vi "Wash Display.vi"(8 "error in (no error)":errorcluster, 11 "Message Queues":T1) -> (0 "error out":errorcluster)   [LabVIEW 2017]
uses:
  support/Message Queue/All Message Queues.ctl
  support/Message Queue/Message Cluster.ctl
  Entry Display Data.ctl
  Position Slider.ctl
  Wash Step Indicators.ctl
  <vilib>/ErrorRing/Error Ring.xnode
  support/Message Queue/Message Queue.lvlib
panel:
  out "Time Eclipse":dbl
  out "Wash Entry Display":bool
  out "Vehicle Position":bool
  out "Air Dry":bool
  out "Tire Shine Foam":bool
  out "Spot Free Rinse":bool
  out "Low Pressure  Wax":bool
  out "High Pressure Wash":bool
  out "Pre-soak":bool
  out "Bug Remover":bool
  out "Under Body Wash":bool
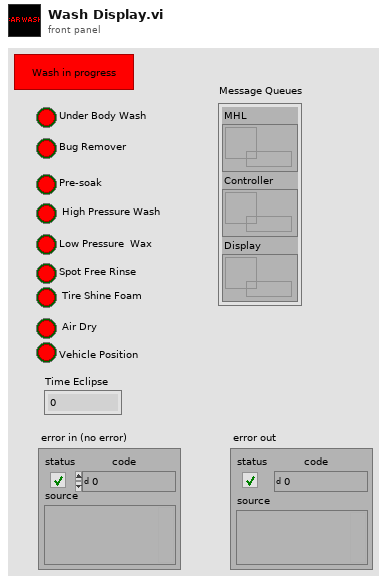
[diagram p1: front panel]
types:
  T1 = typedef "Message Queue.lvlib/All Message Queues.ctl" = cluster{"MHL":refnum<queue>, "Controller":refnum<queue>, "Display":refnum<queue>}
  T2 = typedef "Entry Display Data.ctl" = cluster{"Wash Entry Display":bool, "Car Position Slider":T3, "Wash Display Indicators":T4, "Vehicle Postion":bool}
  T3 = typedef "Position Slider.ctl" = i32
  T4 = typedef "Wash Step Indicators.ctl" = cluster{"Under Body Wash":bool, "Bug Remover":bool, "Pre-soak":bool, " High Pressure Wash":bool, "Low Pressure  Wax":bool, "Spot Free Rinse":bool, " Tire Shine Foam":bool, " Air Dry":bool}
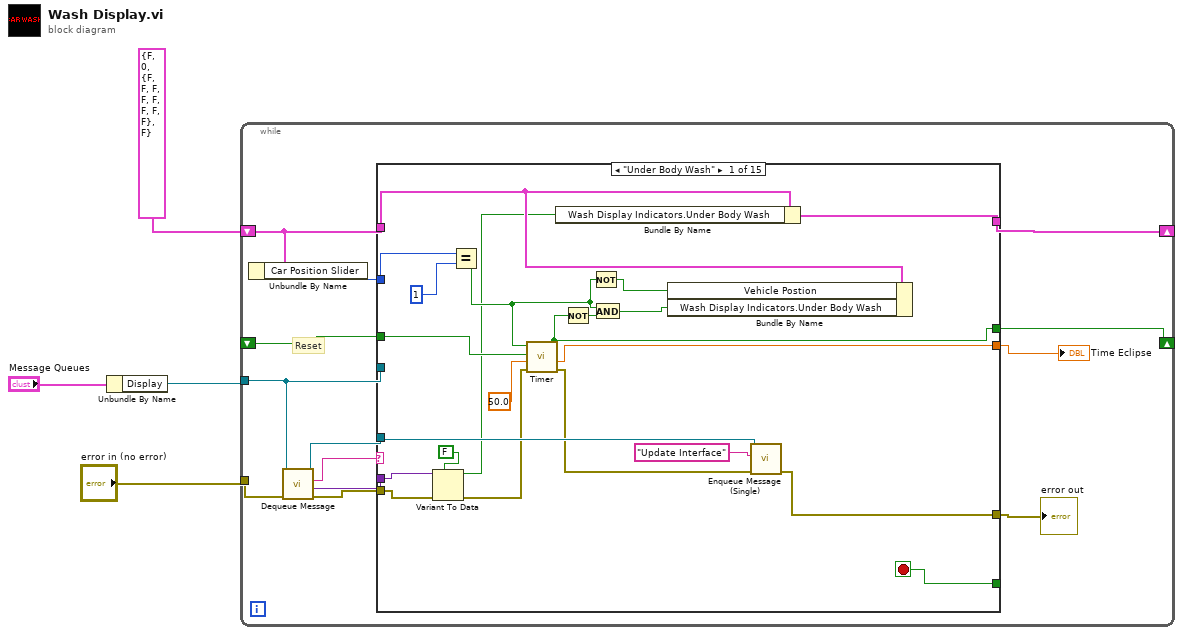
[diagram p0: block diagram]
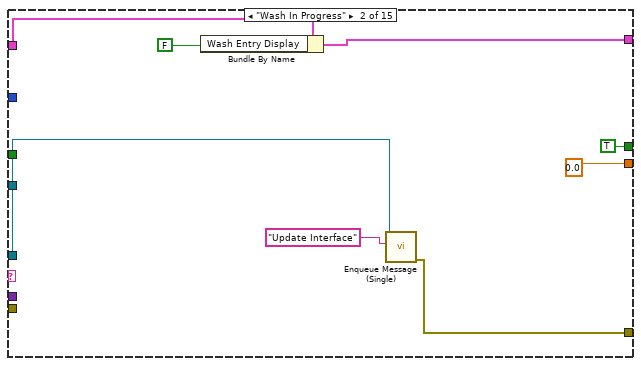
[diagram p2: hidden frame]
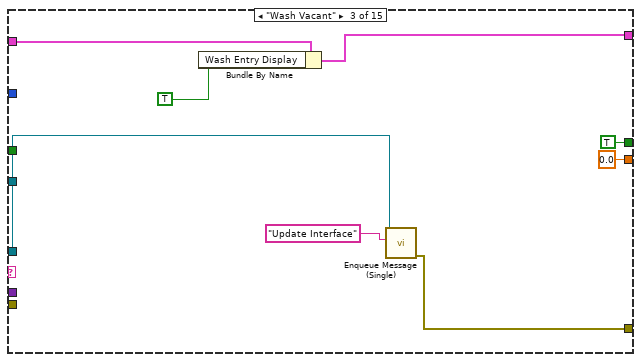
[diagram p3: hidden frame]
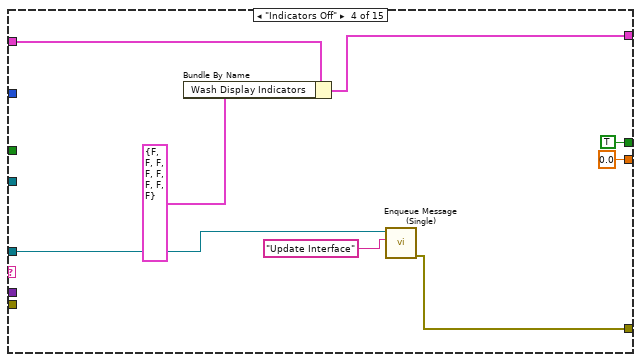
[diagram p4: hidden frame]
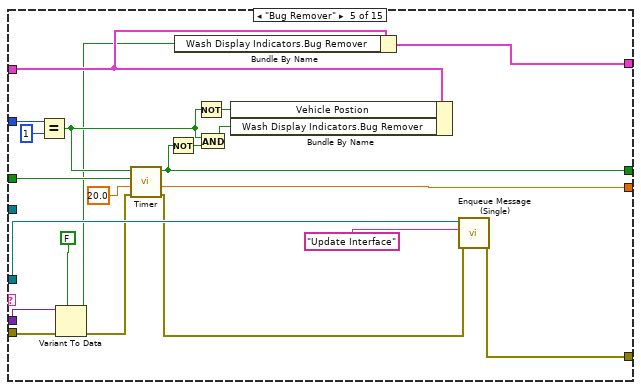
[diagram p5: hidden frame]
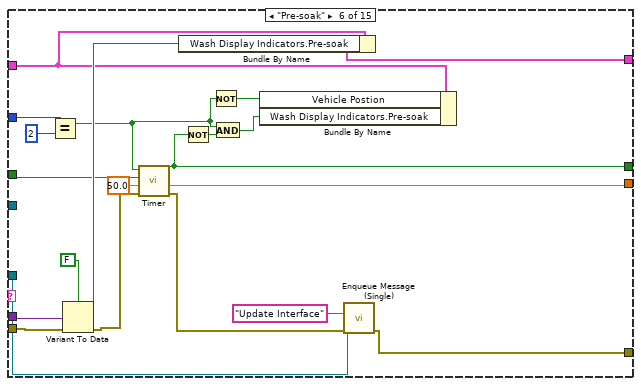
[diagram p6: hidden frame]
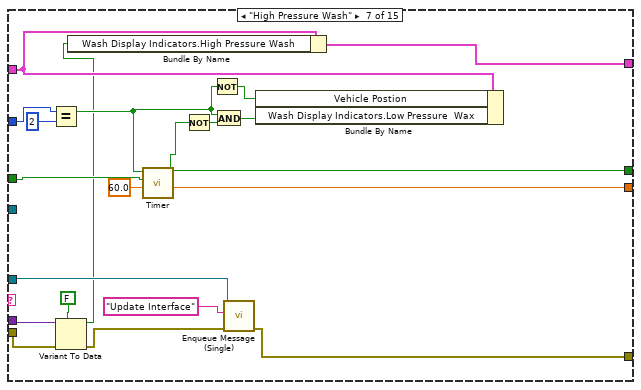
[diagram p7: hidden frame]
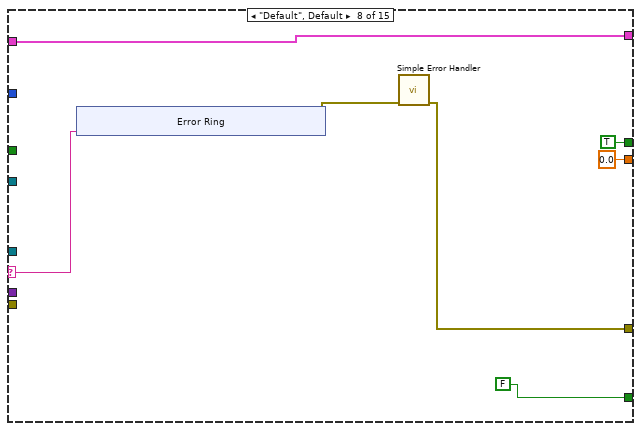
[diagram p8: hidden frame]
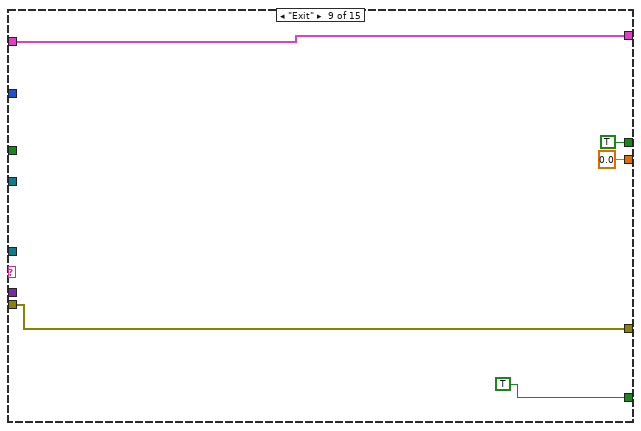
[diagram p9: hidden frame]
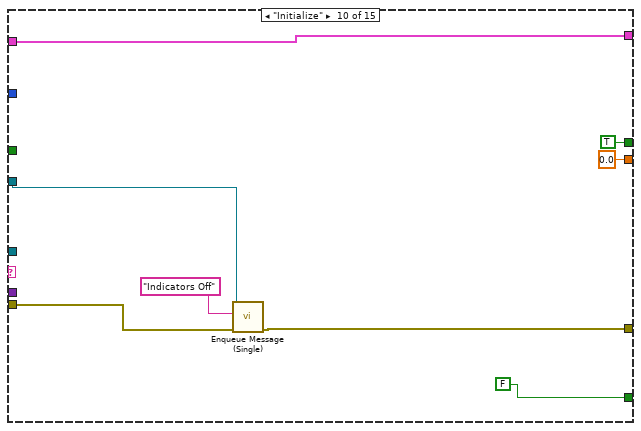
[diagram p10: hidden frame]
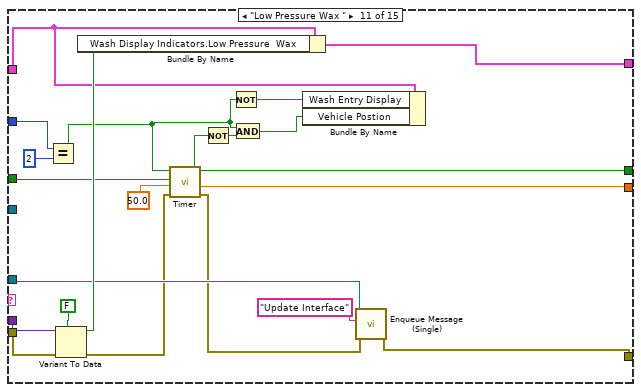
[diagram p11: hidden frame]
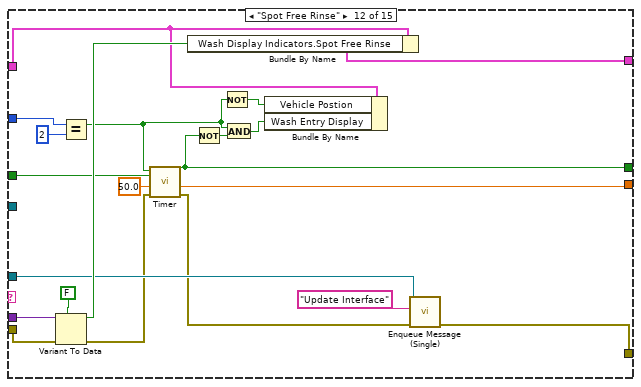
[diagram p12: hidden frame]
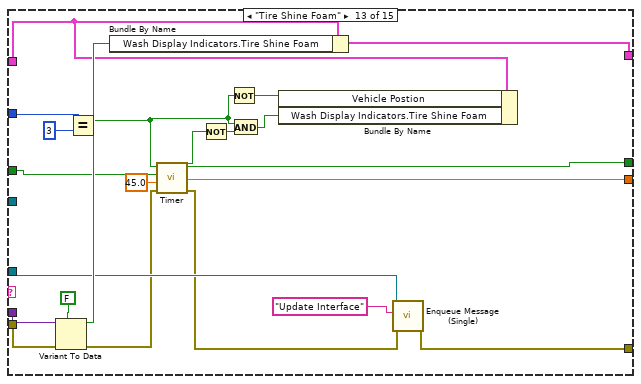
[diagram p13: hidden frame]
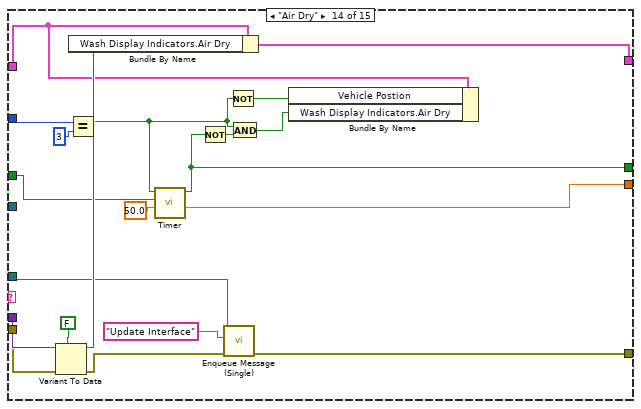
[diagram p14: hidden frame]
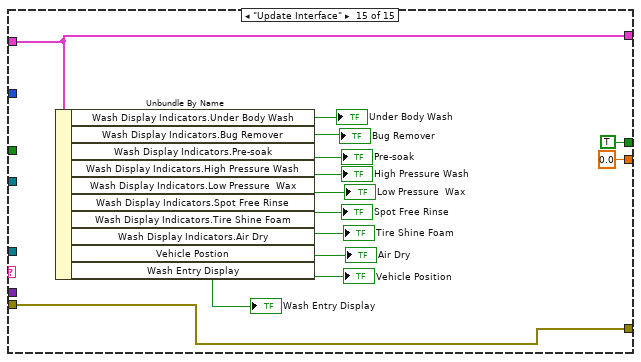
[diagram p15: hidden frame]
diagram:
  n1 = Unbundle By Name("Message Queues") -> ("Display"=w3:refnum<queue>)
  n2 = while {
    tunnel: w3 -> [w12]
    shift-right: [w17] -> _
    shift-left: T2 {"Wash Entry Display"=FALSE, "Car Position Slider"=0, "Wash Display Indicators"={"Under Body Wash"=FALSE, "Bug Remover"=FALSE, "Pre-soak"=FALSE, " High Pressure Wash"=FALSE, "Low Pressure  Wax"=FALSE, "Spot Free Rinse"=FALSE, " Tire Shine Foam"=FALSE, " Air Dry"=FALSE}, "Vehicle Postion"=FALSE} ("Cluster") -> [w10]
    tunnel: "error in (no error)" -> [w11]
    shift-right: [w7] -> _
    shift-left: _ -> [w8]
    stop <- w14 stop-if-true
    # "Reset"
    n3 = Unbundle By Name(w10) -> ("Car Position Slider"=w9:T3)
    n4 = call "Dequeue Message.vi"("error in (no error)"=w11, "Message Queue"=w12) -> ("error out"=w13:errorcluster, "Message Data"=w15:variant, "Message"=w18:string, "dup Message Queue"=w16:refnum<queue>)  [unwired: 6 in]
    n5 = case shown="\"Under Body Wash\"" w18 {
      selector: w18 -> [_ _ _ _ _ _ _ w129 _ _ _ _ _ _ _]
      tunnel: w10 -> [w35 w44 w52 w60 w67 w95 w117 w132 w142 w150 w159 w177 w195 w224 w247]
      tunnel: [w39 w47 w55 w63 w66 w102 w123 w132 w142 w150 w168 w189 w210 w230 w247] -> w17
      tunnel: w16 -> [w38 w46 w54 w62 w82 w101 w122 _ _ _ w167 w188 w209 w229 _]
      tunnel: w15 -> [w24 _ _ _ w84 w105 w125 _ _ _ w171 w192 w213 w233 _]
      tunnel: [_ _ _ _ _ _ _ FALSE TRUE FALSE _ _ _ _ _] -> w14
      tunnel: w13 -> [w22 _ _ _ w80 w99 w120 _ w140 w147 w165 w186 w207 w227 w236]
      tunnel: [w36 w43 w51 w59 w79 w98 w118 w128 w140 w146 w164 w185 w206 w225 w236] -> w5
      tunnel: w12 -> [_ _ _ _ _ _ _ _ _ w145 _ _ _ _ _]
      tunnel: w9 -> [w29 _ _ _ w78 w96 w107 _ _ _ w158 w180 w200 w219 _]
      tunnel: w8 -> [w28 _ _ _ w72 w94 w112 _ _ _ w151 w174 w201 w218 _]
      tunnel: [w25 TRUE ("Time Expired?") TRUE ("Time Expired?") TRUE ("Time Expired?") w71 w87 w110 TRUE ("Time Expired?") TRUE ("Time Expired?") TRUE ("Time Expired?") w154 w172 w198 w216 TRUE ("Time Expired?")] -> w7
      tunnel: [w26 0.0 0.0 ("Elapsed Time") 0.0 ("Elapsed Time") w64 w93 w111 0.0 ("Elapsed Time") 0.0 ("Elapsed Time") 0.0 ("Elapsed Time") w155 w173 w199 w217 0.0 ("Elapsed Time")] -> w6
      frame "Under Body Wash" {
        n6 = Variant To Data(error in=w22, type=FALSE, Variant=w24) -> (data=w21:bool, error out=w20:errorcluster)
        n7 = Equal?(x=w29, y=1) -> (x = y?=w32:bool)
        n8 = call "Timer.vi"("error in"=w20, "Time Limit"=50.0, "Reset"=w28, "Advance Time?"=w32) -> ("error out"=w19:errorcluster, "Elapsed Time"=w26:dbl, "Time Expired?"=w25:bool)  [unwired: 5 in]
        n9 = Bundle By Name(cluster=w35, "Wash Display Indicators.Under Body Wash"=w21) -> (w39:T2)
        n10 = Not(x=w25) -> (.not. x?=w33:bool)
        n11 = Not(x=w32) -> (.not. x?=w27:bool)
        n12 = And(x=w32, y=w33) -> (x .and. y?=w30:bool)
        n13 = Bundle By Name(cluster=w35, "Vehicle Postion"=w27, "Wash Display Indicators.Under Body Wash"=w30) -> ()  [unwired: 1 out]
        n14 = call "Enqueue Message (Single).vi"("error in (no error)"=w19, "Message"="Update Interface", "Message Queue"=w38) -> ("error out"=w36:errorcluster)  [unwired: 7 in, 1 out]
      }
      frame "Wash In Progress" {
        n15 = Bundle By Name(cluster=w44, "Wash Entry Display"=FALSE ("Wash Display Indicators.Under Body Wash")) -> (w47:T2)
        n16 = call "Enqueue Message (Single).vi"("Message"="Update Interface", "Message Queue"=w46) -> ("error out"=w43:errorcluster)  [unwired: 8 in, 1 out]
      }
      frame "Wash Vacant" {
        n17 = Bundle By Name(cluster=w52, "Wash Entry Display"=TRUE ("Wash Display Indicators.Under Body Wash")) -> (w55:T2)
        n18 = call "Enqueue Message (Single).vi"("Message"="Update Interface", "Message Queue"=w54) -> ("error out"=w51:errorcluster)  [unwired: 8 in, 1 out]
      }
      frame "Indicators Off" {
        n19 = Bundle By Name(cluster=w60, "Wash Display Indicators"=T4 {"Under Body Wash"=FALSE, "Bug Remover"=FALSE, "Pre-soak"=FALSE, " High Pressure Wash"=FALSE, "Low Pressure  Wax"=FALSE, "Spot Free Rinse"=FALSE, " Tire Shine Foam"=FALSE, " Air Dry"=FALSE} ("Wash Step Indicators")) -> (w63:T2)
        n20 = call "Enqueue Message (Single).vi"("Message"="Update Interface", "Message Queue"=w62) -> ("error out"=w59:errorcluster)  [unwired: 8 in, 1 out]
      }
      frame "Bug Remover" {
        n21 = Equal?(x=w78, y=1) -> (x = y?=w73:bool)
        n22 = Variant To Data(error in=w80, type=FALSE, Variant=w84) -> (data=w65:bool, error out=w69:errorcluster)
        n23 = call "Timer.vi"("error in"=w69, "Time Limit"=20.0, "Reset"=w72, "Advance Time?"=w73) -> ("error out"=w68:errorcluster, "Elapsed Time"=w64:dbl, "Time Expired?"=w71:bool)  [unwired: 5 in]
        n24 = Not(x=w71) -> (.not. x?=w76:bool)
        n25 = Bundle By Name(cluster=w67, "Wash Display Indicators.Bug Remover"=w65) -> (w66:T2)
        n26 = Not(x=w73) -> (.not. x?=w75:bool)
        n27 = And(x=w73, y=w76) -> (x .and. y?=w74:bool)
        n28 = Bundle By Name(cluster=w67, "Vehicle Postion"=w75, "Wash Display Indicators.Bug Remover"=w74) -> ()  [unwired: 1 out]
        n29 = call "Enqueue Message (Single).vi"("error in (no error)"=w68, "Message"="Update Interface", "Message Queue"=w82) -> ("error out"=w79:errorcluster)  [unwired: 7 in, 1 out]
      }
      frame "Pre-soak" {
        n30 = Equal?(x=w96, y=2) -> (x = y?=w86:bool)
        n31 = Variant To Data(error in=w99, type=FALSE, Variant=w105) -> (data=w104:bool, error out=w92:errorcluster)
        n32 = call "Timer.vi"("error in"=w92, "Time Limit"=50.0, "Reset"=w94, "Advance Time?"=w86) -> ("error out"=w91:errorcluster, "Elapsed Time"=w93:dbl, "Time Expired?"=w87:bool)  [unwired: 5 in]
        n33 = Bundle By Name(cluster=w95, "Wash Display Indicators.Pre-soak"=w104) -> (w102:T2)
        n34 = Not(x=w87) -> (.not. x?=w90:bool)
        n35 = Not(x=w86) -> (.not. x?=w89:bool)
        n36 = And(x=w86, y=w90) -> (x .and. y?=w88:bool)
        n37 = Bundle By Name(cluster=w95, "Vehicle Postion"=w89, "Wash Display Indicators.Pre-soak"=w88) -> ()  [unwired: 1 out]
        n38 = call "Enqueue Message (Single).vi"("error in (no error)"=w91, "Message"="Update Interface", "Message Queue"=w101) -> ("error out"=w98:errorcluster)  [unwired: 7 in, 1 out]
      }
      frame "High Pressure Wash" {
        n39 = Equal?(x=w107, y=2) -> (x = y?=w114:bool)
        n40 = Variant To Data(error in=w120, type=FALSE, Variant=w125) -> (data=w106:bool, error out=w119:errorcluster)
        n41 = Bundle By Name(cluster=w117, "Wash Display Indicators.High Pressure Wash"=w106) -> (w123:T2)
        n42 = call "Timer.vi"("Time Limit"=60.0, "Reset"=w112, "Advance Time?"=w114) -> ("Elapsed Time"=w111:dbl, "Time Expired?"=w110:bool)  [unwired: 6 in, 1 out]
        n43 = Not(x=w110) -> (.not. x?=w115:bool)
        n44 = Not(x=w114) -> (.not. x?=w108:bool)
        n45 = And(x=w114, y=w115) -> (x .and. y?=w109:bool)
        n46 = call "Enqueue Message (Single).vi"("error in (no error)"=w119, "Message"="Update Interface", "Message Queue"=w122) -> ("error out"=w118:errorcluster)  [unwired: 7 in, 1 out]
        n47 = Bundle By Name(cluster=w117, "Vehicle Postion"=w108, "Wash Display Indicators.Low Pressure  Wax"=w109) -> ()  [unwired: 1 out]
      }
      frame "Default", Default {
        n48 = xnode "Error Ring"("parameter 0"=w129) -> ("error out"=w130:errorcluster)
        n49 = call <vilib>:"Simple Error Handler.vi"("error in (no error)"=w130) -> ("error out"=w128:errorcluster)  [unwired: 4 in, 4 out]
      }
      frame "Exit" {
      }
      frame "Initialize" {
        n50 = call "Enqueue Message (Single).vi"("error in (no error)"=w147, "Message"="Indicators Off", "Message Queue"=w145) -> ("error out"=w146:errorcluster)  [unwired: 7 in, 1 out]
      }
      frame "Low Pressure Wax " {
        n51 = Equal?(x=w158, y=2) -> (x = y?=w161:bool)
        n52 = Variant To Data(error in=w165, type=FALSE, Variant=w171) -> (data=w170:bool, error out=w153:errorcluster)
        n53 = Bundle By Name(cluster=w159, "Wash Display Indicators.Low Pressure  Wax"=w170) -> (w168:T2)
        n54 = call "Timer.vi"("error in"=w153, "Time Limit"=50.0, "Reset"=w151, "Advance Time?"=w161) -> ("error out"=w152:errorcluster, "Elapsed Time"=w155:dbl, "Time Expired?"=w154:bool)  [unwired: 5 in]
        n55 = Not(x=w154) -> (.not. x?=w162:bool)
        n56 = Not(x=w161) -> (.not. x?=w157:bool)
        n57 = And(x=w161, y=w162) -> (x .and. y?=w156:bool)
        n58 = Bundle By Name(cluster=w159, "Wash Entry Display"=w157, "Vehicle Postion"=w156) -> ()  [unwired: 1 out]
        n59 = call "Enqueue Message (Single).vi"("error in (no error)"=w152, "Message"="Update Interface", "Message Queue"=w167) -> ("error out"=w164:errorcluster)  [unwired: 7 in, 1 out]
      }
      frame "Spot Free Rinse" {
        n60 = Variant To Data(error in=w186, type=FALSE, Variant=w192) -> (data=w191:bool, error out=w179:errorcluster)
        n61 = Equal?(x=w180, y=2) -> (x = y?=w182:bool)
        n62 = call "Timer.vi"("error in"=w179, "Time Limit"=50.0, "Reset"=w174, "Advance Time?"=w182) -> ("error out"=w178:errorcluster, "Elapsed Time"=w173:dbl, "Time Expired?"=w172:bool)  [unwired: 5 in]
        n63 = Bundle By Name(cluster=w177, "Wash Display Indicators.Spot Free Rinse"=w191) -> (w189:T2)
        n64 = Not(x=w172) -> (.not. x?=w183:bool)
        n65 = Not(x=w182) -> (.not. x?=w176:bool)
        n66 = And(x=w182, y=w183) -> (x .and. y?=w175:bool)
        n67 = Bundle By Name(cluster=w177, "Vehicle Postion"=w176, "Wash Entry Display"=w175) -> ()  [unwired: 1 out]
        n68 = call "Enqueue Message (Single).vi"("error in (no error)"=w178, "Message"="Update Interface", "Message Queue"=w188) -> ("error out"=w185:errorcluster)  [unwired: 7 in, 1 out]
      }
      frame "Tire Shine Foam" {
        n69 = Variant To Data(error in=w207, type=FALSE, Variant=w213) -> (data=w212:bool, error out=w197:errorcluster)
        n70 = Equal?(x=w200, y=3) -> (x = y?=w203:bool)
        n71 = Bundle By Name(cluster=w195, "Wash Display Indicators.Tire Shine Foam"=w212) -> (w210:T2)
        n72 = call "Timer.vi"("error in"=w197, "Time Limit"=45.0, "Reset"=w201, "Advance Time?"=w203) -> ("error out"=w196:errorcluster, "Elapsed Time"=w199:dbl, "Time Expired?"=w198:bool)  [unwired: 5 in]
        n73 = Not(x=w198) -> (.not. x?=w204:bool)
        n74 = Not(x=w203) -> (.not. x?=w193:bool)
        n75 = And(x=w203, y=w204) -> (x .and. y?=w194:bool)
        n76 = Bundle By Name(cluster=w195, "Vehicle Postion"=w193, "Wash Display Indicators.Tire Shine Foam"=w194) -> ()  [unwired: 1 out]
        n77 = call "Enqueue Message (Single).vi"("error in (no error)"=w196, "Message"="Update Interface", "Message Queue"=w209) -> ("error out"=w206:errorcluster)  [unwired: 7 in, 1 out]
      }
      frame "Air Dry" {
        n78 = Variant To Data(error in=w227, type=FALSE, Variant=w233) -> (data=w232:bool, error out=w226:errorcluster)
        n79 = Equal?(x=w219, y=3) -> (x = y?=w221:bool)
        n80 = Bundle By Name(cluster=w224, "Wash Display Indicators.Air Dry"=w232) -> (w230:T2)
        n81 = call "Timer.vi"("Time Limit"=50.0, "Reset"=w218, "Advance Time?"=w221) -> ("Elapsed Time"=w217:dbl, "Time Expired?"=w216:bool)  [unwired: 6 in, 1 out]
        n82 = Not(x=w216) -> (.not. x?=w222:bool)
        n83 = call "Enqueue Message (Single).vi"("error in (no error)"=w226, "Message"="Update Interface", "Message Queue"=w229) -> ("error out"=w225:errorcluster)  [unwired: 7 in, 1 out]
        n84 = Not(x=w221) -> (.not. x?=w215:bool)
        n85 = And(x=w221, y=w222) -> (x .and. y?=w214:bool)
        n86 = Bundle By Name(cluster=w224, "Vehicle Postion"=w215, "Wash Display Indicators.Air Dry"=w214) -> ()  [unwired: 1 out]
      }
      frame "Update Interface" {
        n87 = Unbundle By Name(w247) -> ("Wash Display Indicators.Under Body Wash"=→"Under Body Wash":bool, "Wash Display Indicators.Bug Remover"=→"Bug Remover":bool, "Wash Display Indicators.Pre-soak"=→"Pre-soak":bool, "Wash Display Indicators.High Pressure Wash"=→"High Pressure Wash":bool, "Wash Display Indicators.Low Pressure  Wax"=→"Low Pressure  Wax":bool, "Wash Display Indicators.Spot Free Rinse"=→"Spot Free Rinse":bool, "Wash Display Indicators.Tire Shine Foam"=→"Tire Shine Foam":bool, "Wash Display Indicators.Air Dry"=→"Air Dry":bool, "Vehicle Postion"=→"Vehicle Position":bool, "Wash Entry Display"=→"Wash Entry Display":bool)
      }
    }
    "Time Eclipse" <- w6
    "error out" <- w5
  }
